vi "Get VIs.vi"(8 "error in (no error)":errorcluster) -> (0 "error out":errorcluster, 3 "VIs":refnum<vi>[](array[refnum]))   [LabVIEW 2025, in "Tools.lvlib"]
uses:
  Tools.lvlib
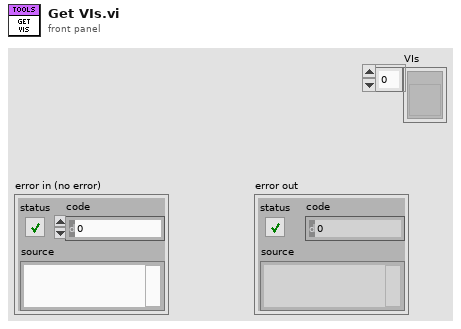
[diagram p1: front panel]
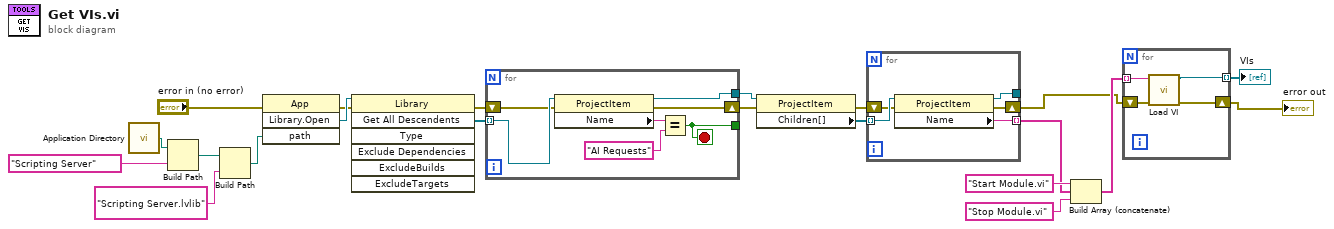
[diagram p0: block diagram]
diagram:
  n1 = call <vilib>:"Application Directory.vi"() -> ("Application Directory"=w14:path)
  n2 = Build Path(base path=w14, name or relative path="Scripting Server" ("format string")) -> (appended path=w16:path)
  n3 = Build Path(base path=w16, name or relative path="Scripting Server.lvlib" ("format string")) -> (appended path=w18:path)
  n4 = invoke class="App" method="Library.Open"(error in="error in (no error)", "path"=w18) -> (error out=w19:errorcluster, "Open Library"=w20:refnum<vi>)  [unwired: 2 in, 2 out]
  n5 = invoke class="Library" method="Get All Descendents"(reference=w20, error in=w19) -> (error out=w11:errorcluster, "All Descendents"=w10:refnum<vi>[])  [unwired: 5 in, 5 out]
  n6 = for {
    tunnel: w10 -> [w28] mode=indexing
    tunnel: [w27] -> w12
    shift-right: [w23] -> w13
    shift-left: w11 -> [w24]
    tunnel: [w22] -> _
    stop <- w22 stop-if-true
    n7 = property class="ProjectItem"(reference=w28, error in=w24) -> (reference out=w27:refnum<vi>, error out=w23:errorcluster, "Name"=w26:string)
    n8 = Equal?(x=w26, y="AI Requests") -> (x = y?=w22:bool)
  }
  n9 = property class="ProjectItem"(reference=w12, error in=w13) -> (error out=w6:errorcluster, "Children[]"=w5:refnum<vi>[])  [unwired: 1 out]
  n10 = for {
    tunnel: w5 -> [w33] mode=indexing
    tunnel: [w32] -> _
    tunnel: [w31] -> w7 mode=indexing
    shift-right: [w29] -> w3
    shift-left: w6 -> [w30]
    n11 = property class="ProjectItem"(reference=w33, error in=w30) -> (reference out=w32:refnum<vi>, error out=w29:errorcluster, "Name"=w31:string)
  }
  n12 = Build Array (concatenate)("Start Module.vi" ("y"), w7, "Stop Module.vi" ("y")) -> (w4:string[])
  n13 = for {
    tunnel: w4 -> [w37] mode=indexing
    shift-right: [w36] -> w2
    shift-left: w3 -> [w35]
    tunnel: [w34] -> w1 mode=indexing
    n14 = call "Load VI.vi"("error in (no error)"=w35, "y"=w37) -> ("error out"=w36:errorcluster, "VI out"=w34:refnum<vi>)  [unwired: 8 in]
  }
  "error out" <- w2
  "VIs" <- w1
